vi "Read MathcadV from file.vi"(8 "error in (no error)":errorcluster, 11 "Path":path) -> (0 "error out":errorcluster, 2 "Variable Clusters out":T1)   [LabVIEW 2012, in "Design Server.lvlib"]
uses:
  Design Server.lvlib
  Variable cluster.ctl
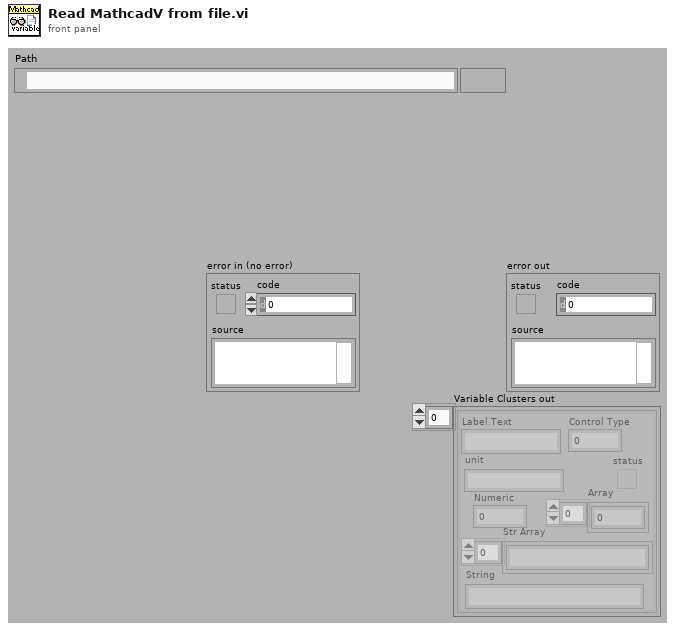
[diagram p1: front panel]
types:
  T1 = typedef "Design Server.lvlib/Variable cluster.ctl" = cluster{"Label.Text":string, "Control Type":u32, "Numeric":dbl, "Array":dbl[], "status":bool, "Str Array":string[], "String":string, "unit":string}[]
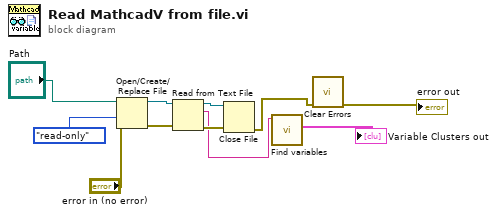
[diagram p0: block diagram]
diagram:
  n1 = Open/Create/Replace File(file path (use dialog)="Path", error in="error in (no error)", access (0:read/write)=enum16{"read/write", "read-only", "write-only"}."read-only") -> (refnum out=w9:refnum<file>, error out=w8:errorcluster)  [unwired: 3 in, 1 out]
  n2 = Read from Text File(file (use dialog)=w9, error in=w8) -> (refnum out=w10:refnum<file>, text=w5:string, error out=w11:errorcluster)  [unwired: 2 in, 1 out]
  n3 = Close File(refnum=w10, error in=w11) -> (error out=w2:errorcluster)  [unwired: 1 out]
  n4 = call "Find variables.vi"("XML"=w5) -> ("Variable Clusters out"=→"Variable Clusters out":T1)  [unwired: 9 in, 1 out]
  n5 = call <vilib>:"Clear Errors.vi"("error in (no error)"=w2) -> ("error out"=→"error out":errorcluster)  [unwired: 6 in]
